vi "test stop notifier.vi"(8 "error in (no error)":errorcluster, 11 "TestCase in":refnum<class "Server Stop Notifier Tests.lvclass">) -> (0 "error out":errorcluster, 3 "TestCase out":refnum<class "Server Stop Notifier Tests.lvclass">)   [LabVIEW 2017, in "Server Stop Notifier Tests.lvclass"]
uses:
  Server Stop Notifier Tests.lvclass
  <vilib>/addons/_JKI Toolkits/VI Tester/TestCase.llb/TestCase.lvclass
  Classes/Server/JSONRPC Server.lvclass
  C:/Program Files (x86)/National Instruments/LabVIEW 2017/vi.lib/addons/_JKI Toolkits/VI Tester/TestCase.llb/TestCase.lvclass
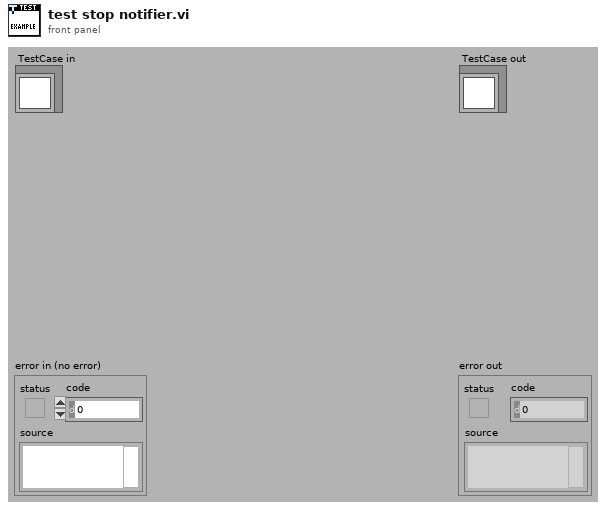
[diagram p1: front panel]
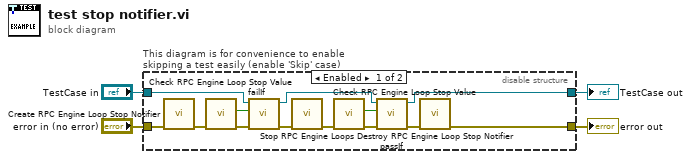
[diagram p0: block diagram]
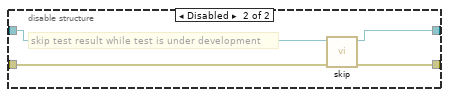
[diagram p2: hidden frame]
diagram:
  n1 = disable-structure "This diagram is for convenience to enable skipping a test easily (enable 'Skip' case)" shown="Enabled" {
    disable-tunnel: "TestCase in" -> [w17 w21]
    disable-tunnel: [w7 w19] -> w1
    disable-tunnel: [w5 w20] -> w3
    disable-tunnel: "error in (no error)" -> [w16 w18]
    frame Enabled {
      n2 = call "Create RPC Engine Loop Stop Notifier.vi"("error in (no error)"=w16) -> ("error out"=w15:errorcluster)  [unwired: 10 in]
      n3 = call "Check RPC Engine Loop Stop Value.vi"("error in (no error)"=w15) -> ("error out"=w14:errorcluster, "stopped?"=w13:bool)  [unwired: 9 in]
      n4 = call-dynamic "failIf.vi"("error in (no error)"=w14, "fail"=w13, "TestCase in"=w17) -> ("error out"=w12:errorcluster, "TestCase out"=w8:refnum<class "Server Stop Notifier Tests.lvclass">)  [unwired: 7 in]
      n5 = call "Stop RPC Engine Loops.vi"("error in (no error)"=w12) -> ("error out"=w11:errorcluster)  [unwired: 10 in]
      n6 = call "Check RPC Engine Loop Stop Value.vi"("error in (no error)"=w11) -> ("error out"=w9:errorcluster, "stopped?"=w10:bool)  [unwired: 9 in]
      n7 = call-dynamic "passIf.vi"("error in (no error)"=w9, "pass"=w10, "TestCase in"=w8) -> ("error out"=w6:errorcluster, "TestCase out"=w7:refnum<class "Server Stop Notifier Tests.lvclass">)  [unwired: 7 in]
      n8 = call "Destroy RPC Engine Loop Stop Notifier.vi"("error in (no error)"=w6) -> ("error out"=w5:errorcluster)  [unwired: 10 in]
    }
    frame Disabled {
      # "skip test result while test is under development"
      n9 = call <vilib>:"skip.vi"("error in (no error)"=w18, "TestCase in"=w21) -> ("error out"=w20:errorcluster, "TestCase out"=w19:refnum<class "Server Stop Notifier Tests.lvclass">)  [unwired: 8 in]
    }
  }
  "error out" <- w3
  "TestCase out" <- w1
